vi "Calculate Average Center.vi"(11 "Gantry Fiducials":dbl[](array[numeric])) -> (3 "XYZTheta":dbl[](array[numeric]))   [LabVIEW 2019, in "Component Tray.lvclass"]
uses:
  Component Tray.lvclass
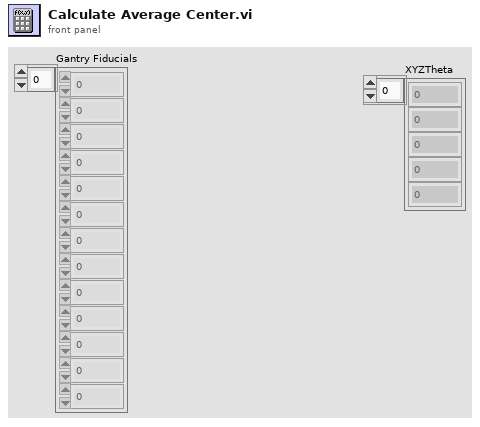
[diagram p1: front panel]
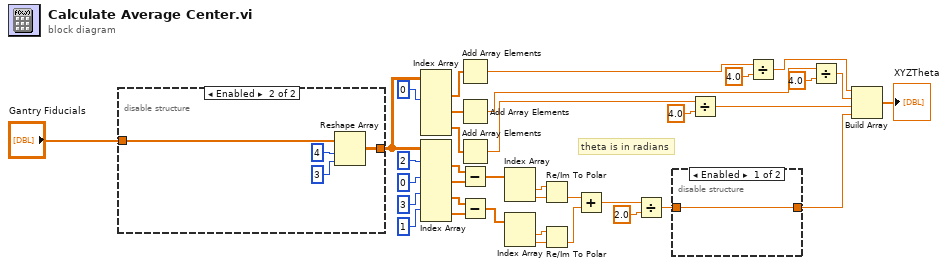
[diagram p0: block diagram]
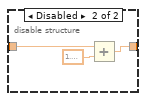
[diagram p2: hidden frame]
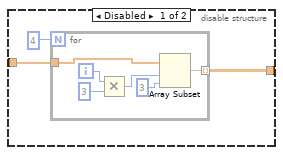
[diagram p3: hidden frame]
diagram:
  # "theta is in radians"
  n1 = disable-structure shown="Enabled" {
    disable-tunnel: "Gantry Fiducials" -> [w39 w49]
    disable-tunnel: [w38 w46] -> w4
    frame Disabled {
      n2 = for {
        N: 4 -> [_]
        tunnel: w39 -> [w41]
        tunnel: [w40] -> w38 mode=indexing
        i -> [w45]
        n3 = Multiply(x=w45, y=3) -> (x*y=w43:i32)
        n4 = Array Subset(array=w41, index=w43, length=3) -> (w40:dbl[])
      }
    }
    frame Enabled {
      n5 = Reshape Array(w49, 4 ("dimension size"), 3 ("dimension size")) -> (w46:dbl[][])
    }
  }
  n6 = Index Array(array=w4, index (col) #1=0 ("disabled index (col)")) -> (element #1=w35:dbl[], element #2=w34:dbl[], element #3=w3:dbl[])  [unwired: 5 in]
  n7 = Index Array(array=w4, index (row) #1=2 ("index (row)"), index (row) #2=0 ("index (row)"), index (row) #3=3 ("index (row)"), index (row) #4=1 ("index (row)")) -> (element #1=w19:dbl[], element #2=w18:dbl[], element #3=w17:dbl[], element #4=w16:dbl[])  [unwired: 4 in]
  n8 = Add Array Elements(numeric array=w35) -> (sum=w33:dbl)
  n9 = Add Array Elements(numeric array=w34) -> (sum=w32:dbl)
  n10 = Add Array Elements(numeric array=w3) -> (sum=w10:dbl)
  n11 = Subtract(x=w19, y=w18) -> (x-y=w29:dbl[])
  n12 = Subtract(x=w17, y=w16) -> (x-y=w28:dbl[])
  n13 = Index Array(array=w29) -> (element #1=w27:dbl, element #2=w26:dbl)  [unwired: 2 in]
  n14 = Index Array(array=w28) -> (element #1=w25:dbl, element #2=w24:dbl)  [unwired: 2 in]
  n15 = Re/Im To Polar(2:w26, 3:w27) -> (0:w23:dbl)  [unwired: 1 out]
  n16 = Re/Im To Polar(2:w24, 3:w25) -> (0:w22:dbl)  [unwired: 1 out]
  n17 = Add(x=w23, y=w22) -> (x+y=w21:dbl)
  n18 = Divide(x=w21, y=2.0) -> (x/y=w2:dbl)
  n19 = disable-structure shown="Enabled" {
    disable-tunnel: w2 -> [w50 w52]
    disable-tunnel: [w50 w51] -> w1
    frame Enabled {
    }
    frame Disabled {
      n20 = Add(x=w52, y=1.5707963267948966) -> (x+y=w51:dbl)
    }
  }
  n21 = Divide(x=w10, y=4.0) -> (x/y=w7:dbl)
  n22 = Divide(x=w33, y=4.0) -> (x/y=w9:dbl)
  n23 = Divide(x=w32, y=4.0) -> (x/y=w8:dbl)
  n24 = Build Array(w9, w8, w7, w1) -> (→"XYZTheta":dbl[])
